vi "TestVirtual4.vi"(0 "reference in":refnum<class "G#BaseClass1.lvclass">, 5 "error in (no error)":errorcluster) -> (14 "reference out":refnum<class "G#BaseClass1.lvclass">, 15 "MethodName":string[](array[string]), 19 "error out":errorcluster)   [LabVIEW 2010, in "G#BaseClass1.lvclass"]
uses:
  G#BaseClass1.lvclass
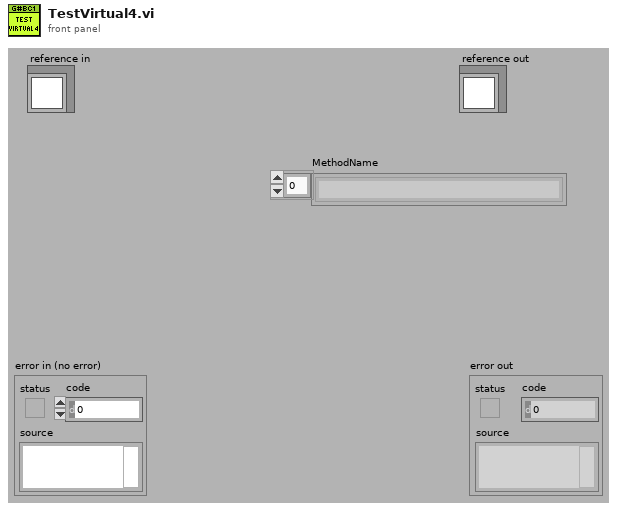
[diagram p1: front panel]
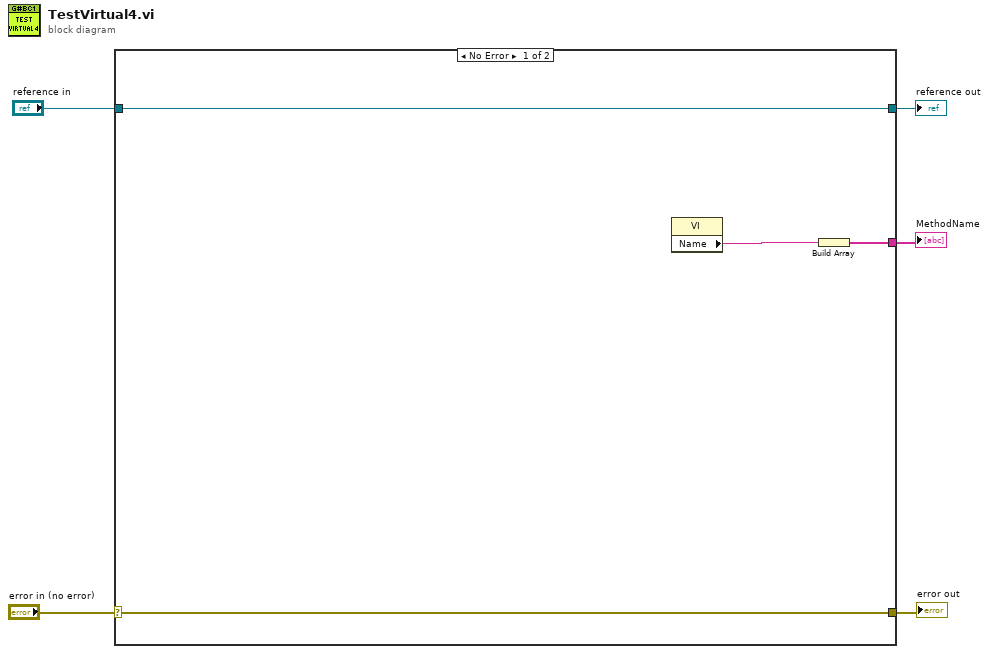
[diagram p0: block diagram]
diagram:
  n1 = case shown="No Error" "error in (no error)" {
    selector: "error in (no error)" -> [w8 w11]
    tunnel: [w8 w11] -> w4
    tunnel: [w9 w10] -> w2
    tunnel: "reference in" -> [w9 w10]
    tunnel: [w7 _] -> w1
    frame No Error {
      n2 = property class="VI"() -> ("Name"=w6:string)  [unwired: 2 in, 2 out]
      n3 = Build Array(w6) -> (w7:string[])
    }
    frame Error {
    }
  }
  "error out" <- w4
  "reference out" <- w2
  "MethodName" <- w1
